vi "Calculate Data Transfer Rate Mbps.vi"(10 "Bytes Sent":i32=1) -> (2 "Mbps":dbl)   [LabVIEW 2023]
uses:
  <vilib>/Rock Robotics/Network Tables/NT Write Number.vi
  <vilib>/ptbypt/NI_PtbyPt.lvlib
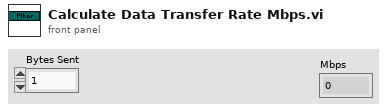
[diagram p1: front panel]
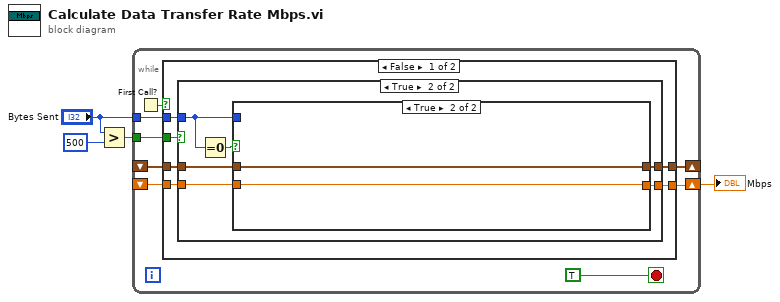
[diagram p0: block diagram]
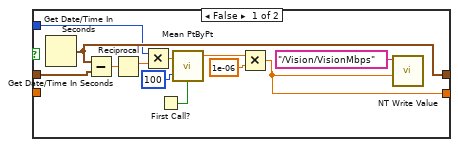
[diagram p3: hidden frame]
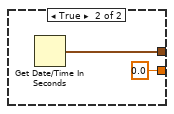
[diagram p4: hidden frame]
diagram:
  n1 = Greater?(x="Bytes Sent", y=500) -> (0:w4:bool)
  n2 = while {
    shift-right: [w11] -> _
    shift-left: _ -> [w12]
    tunnel: "Bytes Sent" -> [w8]
    tunnel: w4 -> [w7]
    shift-right: [w6] -> w1
    shift-left: _ -> [w5]
    stop <- TRUE stop-if-true
    n3 = First Call?() -> (First Call?: T/F=w9:bool)
    n4 = case shown="False" w9 {
      tunnel: w12 -> [w18 _]
      tunnel: [w17 w42] -> w11
      tunnel: w8 -> [w16 _]
      tunnel: w7 -> [w15 _]
      tunnel: [w14 0.0] -> w6
      tunnel: w5 -> [w13 _]
      frame False {
        n5 = case shown="True" w15 {
          tunnel: w18 -> [w20 w26]
          tunnel: [w20 w25] -> w17
          tunnel: w16 -> [_ w24]
          tunnel: [w19 w22] -> w14
          tunnel: w13 -> [w19 w21]
          frame False {
          }
          frame True {
            n6 = Equal To 0?(x=w24) -> (x = 0?=w23:bool)
            n7 = case shown="True" w23 {
              tunnel: w26 -> [w38 w40]
              tunnel: [w37 w40] -> w25
              tunnel: w24 -> [w34 _]
              tunnel: [w28 w39] -> w22
              tunnel: w21 -> [_ w39]
              frame False {
                n8 = Get Date/Time In Seconds() -> ()  [unwired: 1 out]
                n9 = Get Date/Time In Seconds() -> (seconds since 1Jan1904=w37:timestamp)
                n10 = Subtract(x=w37, y=w38) -> (x-y=w36:dbl)
                n11 = Reciprocal(x=w36) -> (1/x=w35:dbl)
                n12 = Multiply(x=w34, y=w35) -> (x*y=w33:dbl)
                n13 = First Call?() -> (First Call?: T/F=w27:bool)
                n14 = call <vilib>:"Mean PtByPt.vi"("x"=w33, "sample length"=100, "initialize"=w27) -> ("mean"=w32:dbl)  [unwired: 1 in, 1 out]
                n15 = Multiply(x=w32, y=1e-06) -> (x*y=w28:dbl)
                n16 = call-poly <vilib>:"NT Write Value.vi"("value"=w28, "name"="/Vision/VisionMbps" ("Name")) -> ()  [unwired: 9 in, 1 out]
              }
              frame True {
              }
            }
          }
        }
      }
      frame True {
        n17 = Get Date/Time In Seconds() -> (seconds since 1Jan1904=w42:timestamp)
      }
    }
  }
  "Mbps" <- w1
